vi "Parse statvfs structure.vi"(8 "error in (no error)":errorcluster, 10 "payload":u8[](array[numeric])) -> (0 "error out":errorcluster, 3 "statvfs":T1 {"f_flag" format="%x"; "f_fsid" format="%x"})   [LabVIEW 2020, in "NI_SFTP.lvlib"]
uses:
  <vilib>/net/SFTP/NI_SFTP.lvlib
  <vilib>/net/SFTP/API/Support/statvfs info.ctl
  3d4df87e-d28e-3fea-a6fc-bfec41c8ef3f.vi
  49ead502-8426-3fe9-bc9b-48340761db3f.vi
  1664b0a4-1b43-3fee-dc93-4db7d934ea3f.vi
  68f9ea6c-24be-3feb-88d5-9e35fa0ee13f.vi
  060cb700-1265-3fbe-d89d-3041409ee23f.vi
  affad1ec-ad30-3fdc-0036-6a11f561bc3f.vi
  a9ba1f64-90ed-3fe8-008e-77b83bb7b13f.vi
  c202c970-adcb-3fe0-c08c-b8c0eb59bc3f.vi
  4a631548-c8db-3fdf-12ab-df936ecde23f.vi
  88fad6a4-8b24-3feb-b034-861508e9e83f.vi
  5fb578c4-87d5-3fef-78d2-e9433cc6d43f.vi
  <vilib>/Bit Manipulation/Network-Order Bytes To Words Poly.vi
  <vilib>/Bit Manipulation/wrappers/Network-Order Bytes To Words/Network-Order Bytes To Words U64.vi
  <vilib>/net/SFTP/Low Level Connection/Low Level Connection.lvclass
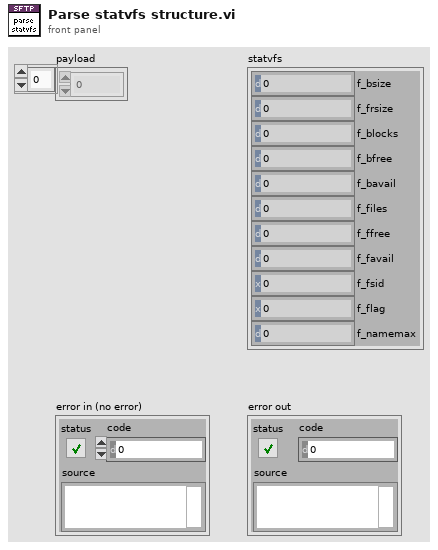
[diagram p1: front panel]
types:
  T1 = typedef "NI_SFTP.lvlib/statvfs info.ctl" = cluster{"f_bsize":u64, "f_frsize":u64, "f_blocks":u64, "f_bfree":u64, "f_bavail":u64, "f_files":u64, "f_ffree":u64, "f_favail":u64, "f_fsid":u64, "f_flag":u64, "f_namemax":u64}
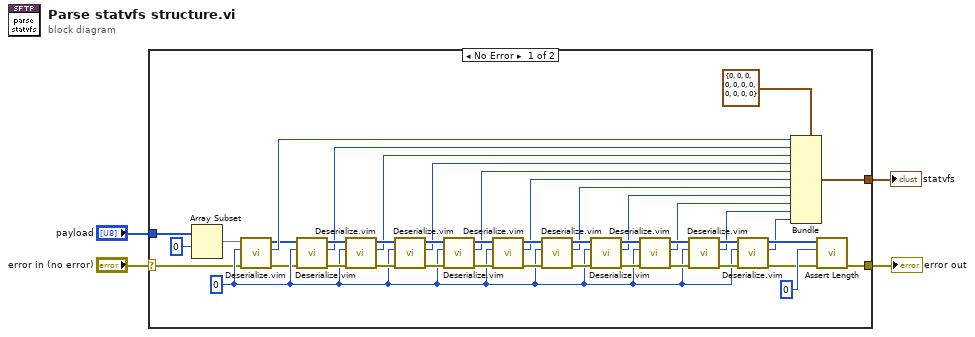
[diagram p0: block diagram]
diagram:
  n1 = case shown="No Error" "error in (no error)" {
    selector: "error in (no error)" -> [w5 w47]
    tunnel: [w46 _] -> w4
    tunnel: [w45 w47] -> w3
    tunnel: "payload" -> [w40 _]
    frame No Error {
      w21 = u64 0
      n2 = Array Subset(array=w40, index=0) -> (w42:u8[])  [unwired: 1 in]
      n3 = call "Deserialize.vim"("error in"=w5, "type"=w21, "bytes"=w42) -> ("error out"=w6:errorcluster, "value"=w8:u64, "remaining bytes"=w7:u8[])  [unwired: 6 in]
      n4 = call "Deserialize.vim"("error in"=w6, "type"=w21, "bytes"=w7) -> ("error out"=w39:errorcluster, "value"=w9:u64, "remaining bytes"=w38:u8[])  [unwired: 6 in]
      n5 = call "Deserialize.vim"("error in"=w39, "type"=w21, "bytes"=w38) -> ("error out"=w24:errorcluster, "value"=w10:u64, "remaining bytes"=w25:u8[])  [unwired: 6 in]
      n6 = call "Deserialize.vim"("error in"=w24, "type"=w21, "bytes"=w25) -> ("error out"=w27:errorcluster, "value"=w11:u64, "remaining bytes"=w26:u8[])  [unwired: 6 in]
      n7 = call "Deserialize.vim"("error in"=w27, "type"=w21, "bytes"=w26) -> ("error out"=w31:errorcluster, "value"=w12:u64, "remaining bytes"=w30:u8[])  [unwired: 6 in]
      n8 = call "Deserialize.vim"("error in"=w31, "type"=w21, "bytes"=w30) -> ("error out"=w28:errorcluster, "value"=w13:u64, "remaining bytes"=w29:u8[])  [unwired: 6 in]
      n9 = call "Deserialize.vim"("error in"=w28, "type"=w21, "bytes"=w29) -> ("error out"=w22:errorcluster, "value"=w14:u64, "remaining bytes"=w23:u8[])  [unwired: 6 in]
      n10 = call "Deserialize.vim"("error in"=w22, "type"=w21, "bytes"=w23) -> ("error out"=w33:errorcluster, "value"=w15:u64, "remaining bytes"=w32:u8[])  [unwired: 6 in]
      n11 = call "Deserialize.vim"("error in"=w33, "type"=w21, "bytes"=w32) -> ("error out"=w37:errorcluster, "value"=w16:u64, "remaining bytes"=w36:u8[])  [unwired: 6 in]
      n12 = call "Deserialize.vim"("error in"=w37, "type"=w21, "bytes"=w36) -> ("error out"=w34:errorcluster, "value"=w17:u64, "remaining bytes"=w35:u8[])  [unwired: 6 in]
      n13 = call "Deserialize.vim"("error in"=w34, "type"=w21, "bytes"=w35) -> ("error out"=w20:errorcluster, "value"=w18:u64, "remaining bytes"=w19:u8[])  [unwired: 6 in]
      n14 = Bundle(cluster=T1 {"f_bsize"=0, "f_frsize"=0, "f_blocks"=0, "f_bfree"=0, "f_bavail"=0, "f_files"=0, "f_ffree"=0, "f_favail"=0, "f_fsid"=0, "f_flag"=0, "f_namemax"=0} ("statvfs@openssh.com reply"), "f_bsize"=w8, "f_frsize"=w9, "f_blocks"=w10, "f_bfree"=w11, "f_bavail"=w12, "f_files"=w13, "f_ffree"=w14, "f_favail"=w15, "f_fsid"=w16, "f_flag"=w17, "f_namemax"=w18) -> (w46:T1)
      n15 = call <vilib>:"Assert Length.vi"("error in"=w20, "asserted length"=u32 0, "string in"=w19) -> ("error out"=w45:errorcluster)  [unwired: 7 in, 1 out]
    }
    frame Error {
    }
  }
  "statvfs" <- w4
  "error out" <- w3
